vi "JoinGroupCommands.vi"(8 "error in (no error)":errorcluster, 9 "Seperator":string[](array[string]), 11 "Msg in":T1) -> (0 "error out":errorcluster, 1 "Seperator out":string=".Channel", 3 "Msg out":T1)   [LabVIEW 2011]
uses:
  DriverMsg.ctl
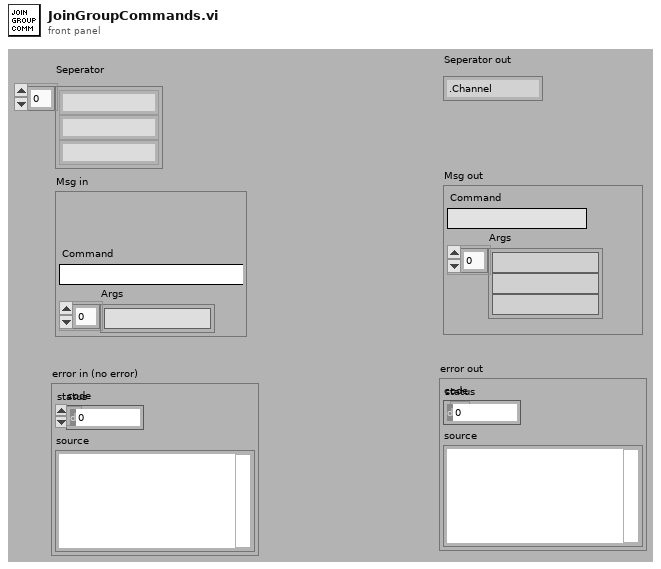
[diagram p1: front panel]
types:
  T1 = typedef "DriverMsg.ctl" = cluster{"Command":string, "Args":string[]}
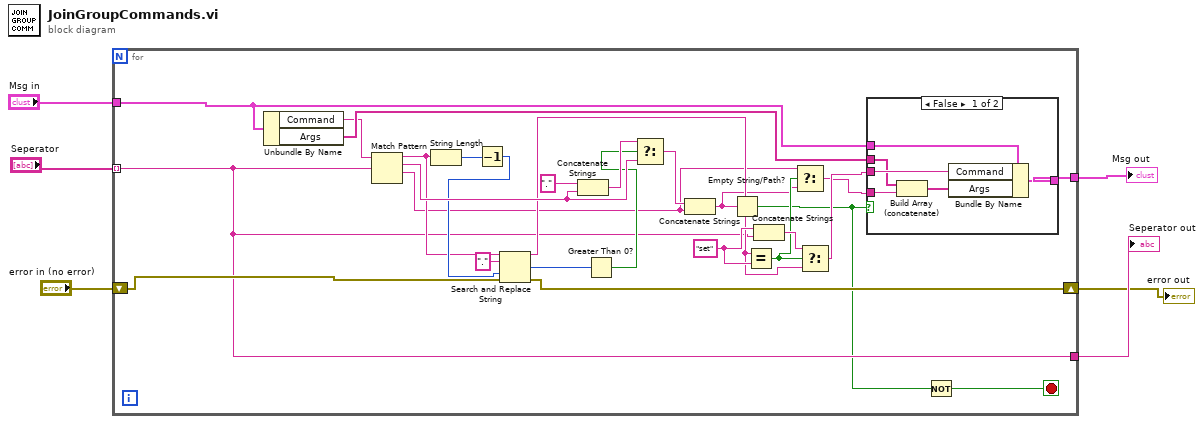
[diagram p0: block diagram]
diagram:
  n1 = for {
    tunnel: [w33] -> w6
    tunnel: [w9] -> w5
    shift-right: [w12] -> w4
    shift-left: "error in (no error)" -> [w11]
    tunnel: "Msg in" -> [w10]
    tunnel: "Seperator" -> [w9] mode=indexing
    stop <- w7 stop-if-true
    w20 = "set" ("y")
    n2 = Unbundle By Name(w10) -> ("Command"=w31:string, "Args"=w32:string[])
    n3 = Match Pattern(string=w31, regular expression=w9) -> (before substring=w21:string, match substring=w28:string, after substring=w15:string)  [unwired: 1 in, 1 out]
    n4 = String Length(string=w21) -> (length=w30:i32)
    n5 = Decrement(x=w30) -> (x-1=w25:i32)
    n6 = Search and Replace String(input string=w21, search string=".", offset=w25, error in=w11) -> (result string=w19:string, number of replacements=w24:i32, error out=w12:errorcluster)  [unwired: 4 in, 1 out]
    n7 = Concatenate Strings("." ("x"), w28) -> (w29:string)
    n8 = Greater Than 0?(x=w24) -> (x > 0?=w23:bool)
    n9 = Select(t=w29, s=w23, f=w28) -> (s? t:f=w27:string)
    n10 = Concatenate Strings(w27, w15) -> (w14:string)
    n11 = Empty String/Path?(string/path=w14) -> (empty?=w8:bool)
    n12 = Equal?(x=w19, y=w20) -> (x = y?=w16:bool)
    n13 = Concatenate Strings(w20, w9) -> (w17:string)
    n14 = Select(t=w15, s=w16, f=w14) -> (s? t:f=w13:string)
    n15 = Select(t=w17, s=w16, f=w19) -> (s? t:f=w18:string)
    n16 = case shown="False" w8 {
      tunnel: w10 -> [w39 w40]
      tunnel: [w38 w40] -> w33
      tunnel: w18 -> [w37 _]
      tunnel: w32 -> [w36 _]
      tunnel: w13 -> [w34 _]
      frame False {
        n17 = Build Array (concatenate)(w36, w34) -> (w35:string[])
        n18 = Bundle By Name(cluster=w39, "Command"=w37, "Args"=w35) -> (w38:T1)
      }
      frame True {
      }
    }
    n19 = Not(x=w8) -> (.not. x?=w7:bool)
  }
  "Msg out" <- w6
  "Seperator out" <- w5
  "error out" <- w4
